vi "PalardyPI.vi"(8 "integral_cap":dbl, 9 "gainset":cluster{"kp":dbl, "ki":dbl, "kd":dbl}, 10 "goal":dbl, 11 "sensor":dbl) -> (3 "motor":dbl)   [LabVIEW 2012]
panel:
  out "error":dbl
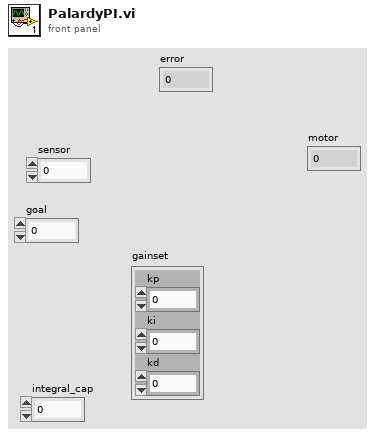
[diagram p1: front panel]
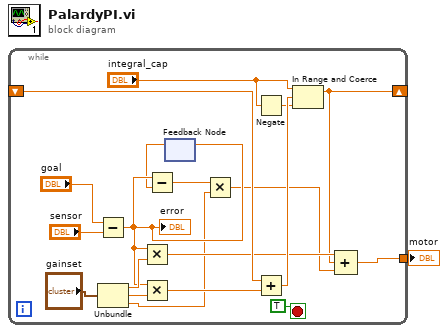
[diagram p0: block diagram]
diagram:
  n1 = while {
    shift-right: [w13] -> _
    shift-left: _ -> [w19]
    tunnel: [w9] -> w1
    stop <- TRUE stop-if-true
    n2 = Subtract(x="goal", y="sensor") -> (x-y=w6:dbl)
    "error" <- w6
    n3 = Unbundle("gainset") -> ("kp"=w11:dbl, "ki"=w10:dbl, "kd"=w3:dbl)
    n4 = Multiply(x=w6, y=w11) -> (x*y=w14:dbl)
    n5 = Multiply(x=w6, y=w10) -> (x*y=w18:dbl)
    n6 = feedback-in #1(w6) -> ()
    n7 = feedback #1() -> (w5:dbl)  [unwired: 1 in]
    n8 = Subtract(x=w6, y=w5) -> (x-y=w4:dbl)
    n9 = Multiply(x=w4, y=w3) -> (x*y=w2:dbl)
    n10 = Negate(x="integral_cap") -> (-x=w16:dbl)
    n11 = Add(x=w19, y=w18) -> (x+y=w17:dbl)
    n12 = In Range and Coerce(upper limit="integral_cap", x=w17, lower limit=w16) -> (coerced(x)=w13:dbl)  [unwired: 1 out]
    n13 = Compound Arithmetic op=ADD(w14, w13, w2) -> (w9:dbl)
  }
  "motor" <- w1
